vi "Destroy.vi"(8 "error in (no error)":errorcluster, 11 "Messages Composite View In":refnum<class "Messages Composite View.lvclass">) -> (0 "error out":errorcluster)   [LabVIEW 2020, in "Messages Composite View.lvclass"]
uses:
  Messages Composite View.lvclass
  Messages Composite View.lvclass/Messages Composite View.ctl
  Debug View/Debug View.lvclass
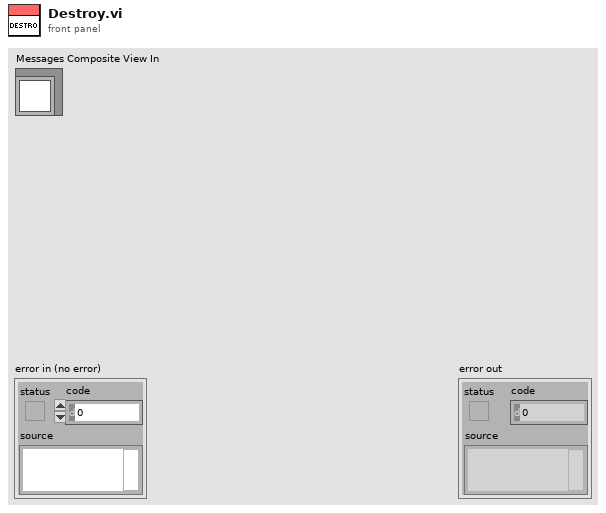
[diagram p1: front panel]
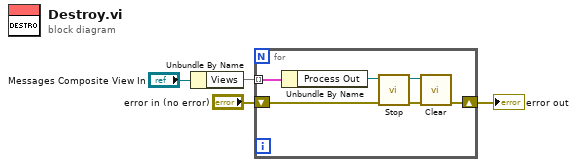
[diagram p0: block diagram]
diagram:
  n1 = Unbundle By Name("Messages Composite View In") -> ("Views"=w3:map{string, refnum<class "Debug View.lvclass">})
  n2 = for {
    tunnel: w3 -> [w10] mode=indexing
    shift-right: [w5] -> w2
    shift-left: "error in (no error)" -> [w6]
    n3 = Unbundle By Name(w10) -> ("Process Out"=w7:refnum<class "Debug View.lvclass">)
    n4 = call "Stop.vi"("error in (no error)"=w6, "Process In"=w7) -> ("error out"=w8:errorcluster, "Process Out"=w9:refnum<class "Debug View.lvclass">)  [unwired: 8 in]
    n5 = call-dynamic "Clear.vi"("error in (no error)"=w8, "Debug View In"=w9) -> ("error out"=w5:errorcluster)  [unwired: 9 in]
  }
  "error out" <- w2
